vi "Analyse.vi"(8 "error in (no error)":errorcluster, 11 "WelcomeHandler MsgPack in":refnum<class "WelcomeHandler MsgPack.lvclass">) -> (0 "error out":errorcluster, 3 "WelcomeHandler MsgPack out":refnum<class "WelcomeHandler MsgPack.lvclass">)   [LabVIEW 2020, in "wamplv.lvlib" / "WelcomeHandler MsgPack.lvclass"]
uses:
  WelcomeHandler MsgPack.lvclass
  WelcomeHandler MsgPack.lvclass/WelcomeHandler MsgPack.ctl
  MessagePack/MessagePackNumeric/MessagePackNumeric.lvclass
  3e4b6e4e-4466-430a-b6e5-9bd36c73e74d.vi
  SerialisedMessages/MsgPackMessage/WampMessage MsgPack.lvclass
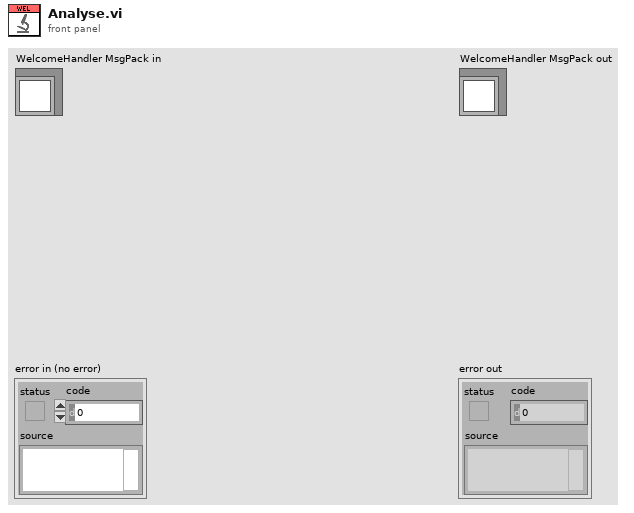
[diagram p1: front panel]
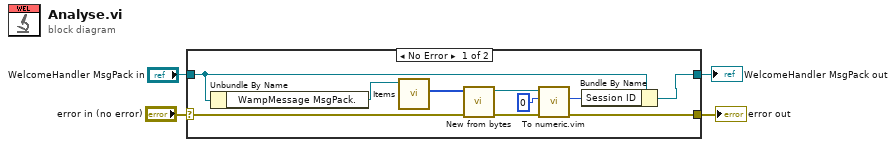
[diagram p0: block diagram]
diagram:
  n1 = case shown="No Error" "error in (no error)" {
    selector: "error in (no error)" -> [w5 w15]
    tunnel: "WelcomeHandler MsgPack in" -> [w6 w16]
    tunnel: [w10 w16] -> w2
    tunnel: [w8 w15] -> w1
    frame No Error {
      n2 = Unbundle By Name(w6) -> ("WampMessage MsgPack."=w7:refnum<class "WampMessage MsgPack.lvclass">)
      n3 = call-dynamic "Items.vi"("MsgPackMessage in"=w7) -> ("Bytes"=w11:u8[])  [unwired: 9 in, 1 out]
      n4 = call "New from bytes.vi"("error in (no error)"=w5, "Bytes"=w11) -> ("error out"=w13:errorcluster, "MessagePackNumeric out"=w14:refnum<class "MessagePackNumeric.lvclass">)  [unwired: 6 in, 2 out]
      n5 = call "To numeric.vim"("error in (no error)"=w13, "Numeric Type"=u64 0, "MessagePackNumeric in"=w14) -> ("error out"=w8:errorcluster, "Reult"=w9:u64)  [unwired: 6 in, 1 out]
      n6 = Bundle By Name(cluster=w6, "Session ID"=w9) -> (w10:refnum<class "WelcomeHandler MsgPack.lvclass">)
    }
    frame Error {
    }
  }
  "error out" <- w1
  "WelcomeHandler MsgPack out" <- w2
